vi "SAPI_Speak_Text_String_SubVI.vi"(4 "Purge other pending text? (F)":bool, 5 "XML? (auto-detect)":T1, 6 "Wait for completion? (F)":bool, 7 "Speak Punctuation (F)":bool, 8 "error in (no error)":errorcluster, 9 "Persist any SAPI settings found in XML (F)":bool, 10 "Text to speak":string, 11 "speech object references":T2) -> (0 "error out":errorcluster, 3 "speech object references (out)":T2)   [LabVIEW 2012]
doc: "Use the current SAPI voice settings to speak the text string wired to the Text input."
uses:
  Controls/Speech object references.ctl
  Controls/SAPI_Speak_Method_XML_Flag_Enum.ctl
  SAPI.TTS.lvlib
panel:
  # "Use the current SAPI voice settings to speak\nthe text string wired to the Text input."
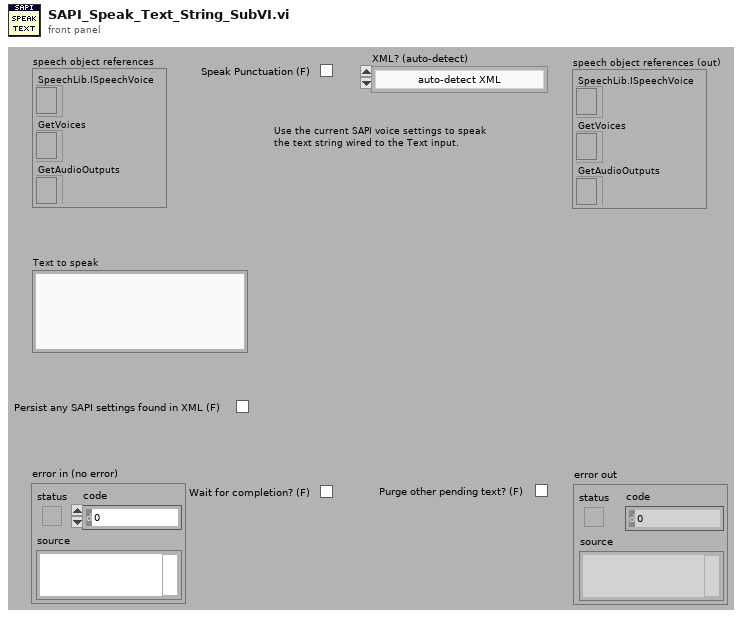
[diagram p1: front panel]
types:
  T1 = typedef "SAPI_Speak_Method_XML_Flag_Enum.ctl" = enum16{"auto-detect XML", "always treat input as XML", "never treat input as XML"}
  T2 = typedef "SAPI.TTS.lvlib/Speech object references.ctl" = cluster{"SpeechLib.ISpeechVoice":refnum<k7>, "GetVoices":refnum<k7>, "GetAudioOutputs":refnum<k7>}
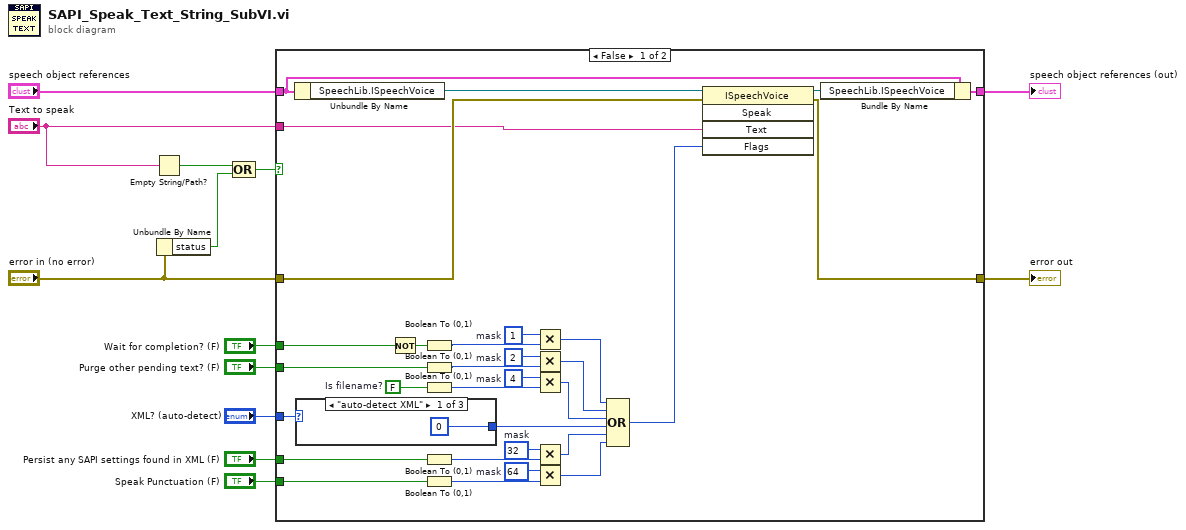
[diagram p0: block diagram]
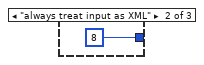
[diagram p2: hidden frame]
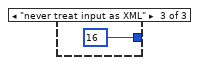
[diagram p3: hidden frame]
diagram:
  n1 = Empty String/Path?(string/path="Text to speak") -> (empty?=w9:bool)
  n2 = Unbundle By Name("error in (no error)") -> ("status"=w8:bool)
  n3 = Compound Arithmetic op=OR(w9, w8) -> (w2:bool)
  n4 = case shown="False" w2 {
    tunnel: "speech object references" -> [w44 w48]
    tunnel: [w43 w49] -> w12
    tunnel: [w42 w48] -> w11
    tunnel: "error in (no error)" -> [w41 w49]
    tunnel: "Wait for completion? (F)" -> [w39 _]
    tunnel: "Speak Punctuation (F)" -> [w37 _]
    tunnel: "Persist any SAPI settings found in XML (F)" -> [w36 _]
    tunnel: "Purge other pending text? (F)" -> [w35 _]
    tunnel: "XML? (auto-detect)" -> [w20 _]
    tunnel: "Text to speak" -> [w17 _]
    frame False {
      w14 = FALSE  # Is filename?
      w30 = 64  # mask
      w31 = 32  # mask
      w32 = 4  # mask
      w33 = 2  # mask
      w40 = 1  # mask
      n5 = Unbundle By Name(w44) -> ("SpeechLib.ISpeechVoice"=w16:refnum<k7>)
      n6 = case shown="\"auto-detect XML\"" w20 {
        tunnel: [0 8 16] -> w19
        frame "auto-detect XML" {
        }
        frame "always treat input as XML" {
        }
        frame "never treat input as XML" {
        }
      }
      n7 = Not(x=w39) -> (.not. x?=w38:bool)
      n8 = Boolean To (0,1)(Boolean=w38) -> (0, 1=w34:i16)
      n9 = Boolean To (0,1)(Boolean=w35) -> (0, 1=w26:i16)
      n10 = Boolean To (0,1)(Boolean=w14) -> (0, 1=w27:i16)
      n11 = Boolean To (0,1)(Boolean=w36) -> (0, 1=w28:i16)
      n12 = Boolean To (0,1)(Boolean=w37) -> (0, 1=w29:i16)
      n13 = Multiply(x=w40, y=w34) -> (x*y=w25:i32)
      n14 = Multiply(x=w33, y=w26) -> (x*y=w24:i32)
      n15 = Multiply(x=w32, y=w27) -> (x*y=w23:i32)
      n16 = Multiply(x=w31, y=w28) -> (x*y=w22:i32)
      n17 = Multiply(x=w30, y=w29) -> (x*y=w18:i32)
      n18 = Compound Arithmetic op=OR(w25, w24, w23, w19, w22, w18) -> (w21:i32)
      n19 = invoke class="ISpeechVoice" method="Speak"(reference=w16, error in=w41, "Text"=w17, "Flags"=w21) -> (reference out=w15:refnum<k7>, error out=w43:errorcluster)  [unwired: 1 in, 3 out]
      n20 = Bundle By Name(cluster=w44, "SpeechLib.ISpeechVoice"=w15) -> (w42:T2)
    }
    frame True {
    }
  }
  "error out" <- w12
  "speech object references (out)" <- w11
